vi "EvaluateAuthorizationExpression.vi"(8 "ErrorIn":errorcluster, 10 "Expression":string, 11 "ReferenceIn":refnum<class "IAuthorization.lvclass">) -> (0 "ErrorOut":errorcluster, 1 "Result":T1, 2 "Pass":bool, 3 "ReferenceIn":refnum<class "IAuthorization.lvclass">)   [LabVIEW 2021, in "IAuthorization.lvclass"]
uses:
  IAuthorization.lvclass
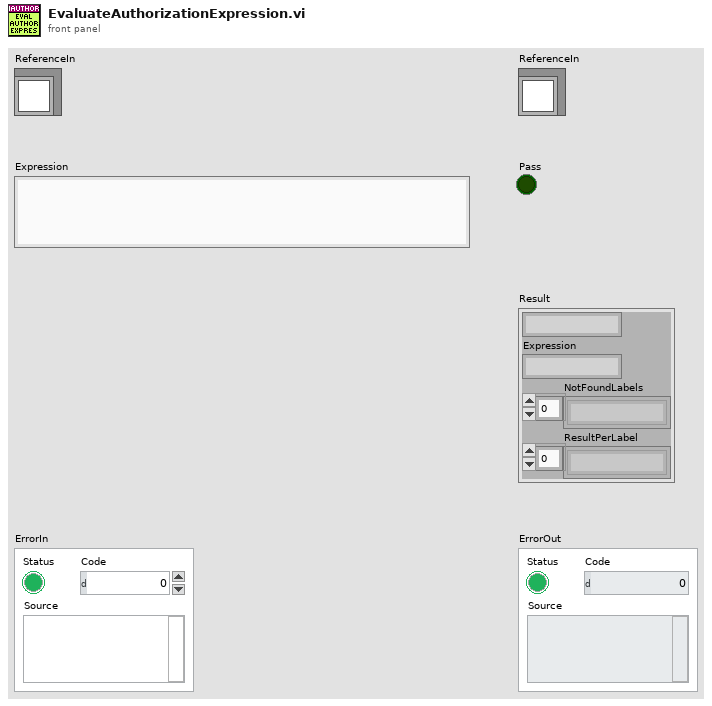
[diagram p1: front panel]
types:
  T1 = cluster{string, "Expression":string, "NotFoundLabels":string[], "ResultPerLabel":string[]}
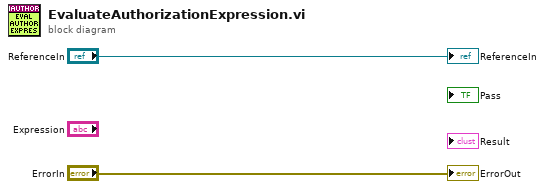
[diagram p0: block diagram]
diagram:
  "ErrorOut" <- "ErrorIn"
  "ReferenceIn" <- "ReferenceIn"
